vi "3457A_REAR_INPUT.vi"(8 "error in (no error)":errorcluster) -> (0 "error out":errorcluster)   [LabVIEW 2020]
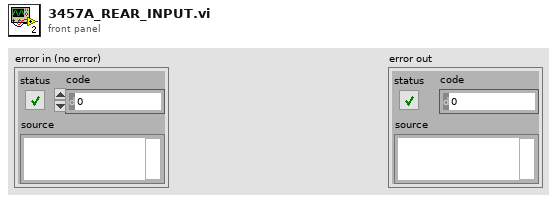
[diagram p1: front panel]
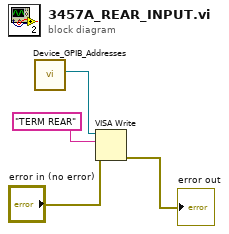
[diagram p0: block diagram]
diagram:
  n1 = call "Device_GPIB_Addresses.vi"() -> ("HP 3457A Address"=w3:refnum<visa-resource-name>)  [unwired: 9 in, 2 out]
  n2 = VISA Write(VISA resource name=w3, write buffer="TERM REAR", error in (no error)="error in (no error)") -> (error out=→"error out":errorcluster)  [unwired: 2 out]
